vi "Clear Stack.vi"(8 "error in (no error)":errorcluster caption="错误输入（无错误）", 11 "Stack 输入":refnum<class "Stack.lvclass"> caption="DNL_LabVIEW Object in") -> (0 "error out":errorcluster caption="错误输出", 3 "Stack 输出":refnum<class "Stack.lvclass"> caption="DNL_LabVIEW Object out")   [LabVIEW 2011, in "Stack.lvclass"]
uses:
  Stack.lvclass
  Stack.lvclass/Stack.ctl
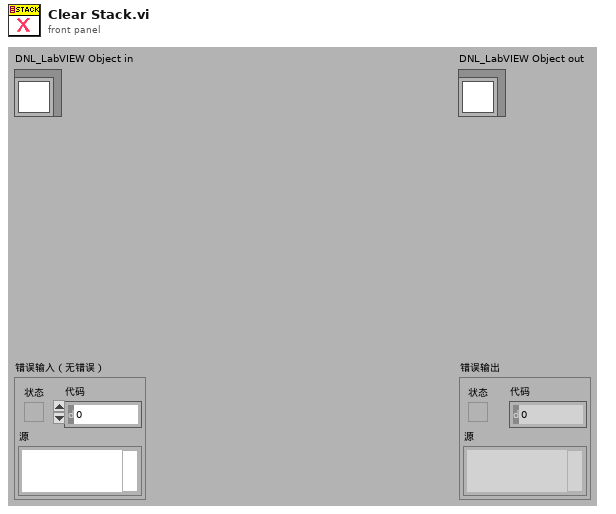
[diagram p1: front panel]
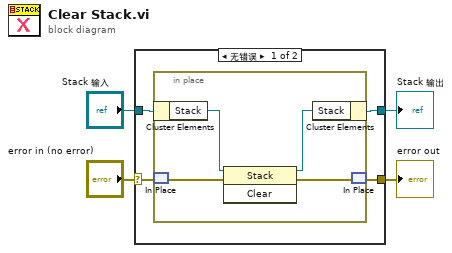
[diagram p0: block diagram]
diagram:
  n1 = case shown="无错误" "error in (no error)" {
    selector: "error in (no error)" -> [w7 w14]
    tunnel: [w6 w14] -> w3
    tunnel: [w5 w13] -> w1
    tunnel: "Stack 输入" -> [w8 w13]
    frame No Error {
      n2 = in-place {
        n3 = in-place-cluster #1(w8) -> ("Stack"=w12:refnum<k24>)
        n4 = in-place-match #2(w7) -> (w10:errorcluster)
        n5 = invoke class="Stack" method="Clear"(reference=w12, error in=w10) -> (reference out=w11:refnum<k24>, error out=w9:errorcluster)  [unwired: 1 in, 1 out]
        n6 = in-place-cluster #1("Stack"=w11) -> (w5:refnum<class "Stack.lvclass">)
        n7 = in-place-match #2(w9) -> (w6:errorcluster)
      }
    }
    frame Error {
    }
  }
  "error out" <- w3
  "Stack 输出" <- w1
